vi "air temp subvi remote.vi"(0 "Boolean in":refnum<vi>, 1 "reference 3":refnum<vi>, 2 "reference 11":refnum<vi>, 3 "reference 4":refnum<vi>, 4 "reference 10":refnum<vi>, 5 "reference 5":refnum<vi>, 6 "reference 6":refnum<vi>, 8 "reference 12":refnum<vi>, 9 "reference 7":refnum<vi>, 10 "reference 2":refnum<vi>, 11 "reference 8":refnum<vi>, 12 "reference":refnum<vi>, 13 "reference 9":refnum<vi>, 14 "reference 14":refnum<vi>, 16 "Numeric":dbl) -> ()   [LabVIEW 2018]
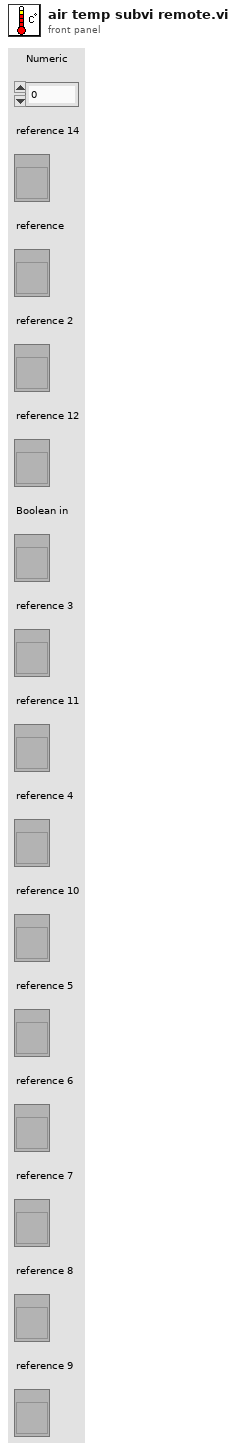
[diagram p1: front panel]
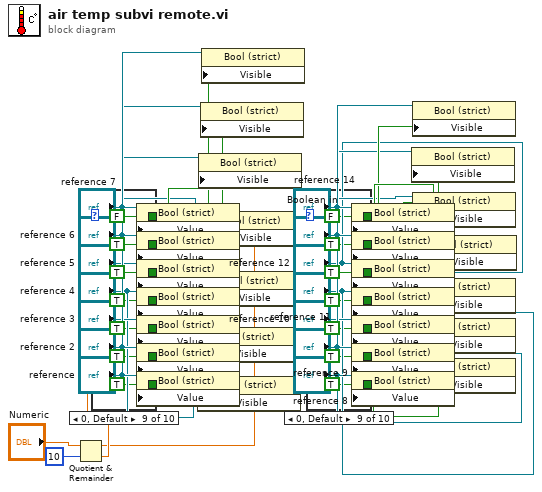
[diagram p0: block diagram]
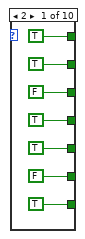
[diagram p2: hidden frame]
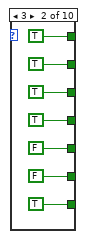
[diagram p3: hidden frame]
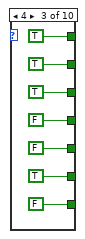
[diagram p4: hidden frame]
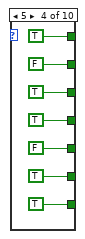
[diagram p5: hidden frame]
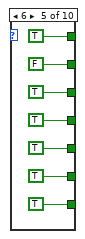
[diagram p6: hidden frame]
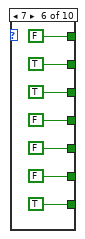
[diagram p7: hidden frame]
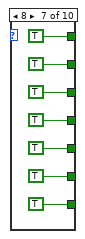
[diagram p8: hidden frame]
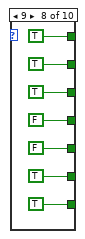
[diagram p9: hidden frame]
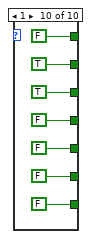
[diagram p10: hidden frame]
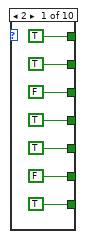
[diagram p11: hidden frame]
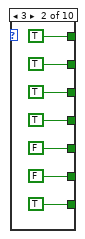
[diagram p12: hidden frame]
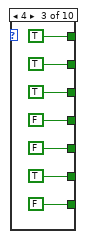
[diagram p13: hidden frame]
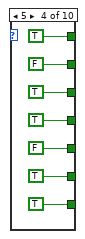
[diagram p14: hidden frame]
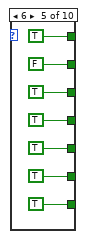
[diagram p15: hidden frame]
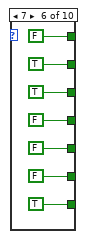
[diagram p16: hidden frame]
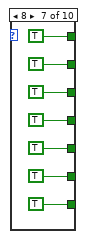
[diagram p17: hidden frame]
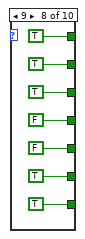
[diagram p18: hidden frame]
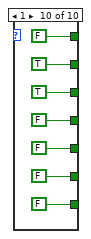
[diagram p19: hidden frame]
diagram:
  n1 = Quotient & Remainder(x="Numeric", y=10) -> (x-y*floor(x/y)=w16:dbl, floor(x/y)=w17:dbl)
  n2 = case shown="0, Default" w17 {
    tunnel: [TRUE TRUE FALSE TRUE TRUE TRUE TRUE TRUE TRUE FALSE] -> w25
    tunnel: [FALSE FALSE TRUE TRUE TRUE FALSE TRUE TRUE TRUE FALSE] -> w26
    tunnel: [TRUE FALSE FALSE FALSE TRUE FALSE TRUE FALSE TRUE FALSE] -> w27
    tunnel: [TRUE TRUE FALSE TRUE TRUE FALSE TRUE FALSE TRUE FALSE] -> w28
    tunnel: [FALSE TRUE TRUE TRUE TRUE TRUE TRUE TRUE TRUE TRUE] -> w29
    tunnel: [TRUE TRUE TRUE FALSE FALSE TRUE TRUE TRUE TRUE TRUE] -> w30
    tunnel: [TRUE TRUE TRUE TRUE TRUE FALSE TRUE TRUE FALSE FALSE] -> w31
    frame 2 {
    }
    frame 3 {
    }
    frame 4 {
    }
    frame 5 {
    }
    frame 6 {
    }
    frame 7 {
    }
    frame 8 {
    }
    frame 9 {
    }
    frame 0, Default {
    }
    frame 1 {
    }
  }
  n3 = property class="Bool (strict)"(reference="reference 7", "Value"=w31) -> ()  [unwired: 1 in, 2 out]
  n4 = property class="Bool (strict)"(reference="reference 6", "Value"=w30) -> ()  [unwired: 1 in, 2 out]
  n5 = property class="Bool (strict)"(reference="reference 5", "Value"=w29) -> ()  [unwired: 1 in, 2 out]
  n6 = property class="Bool (strict)"(reference="reference 4", "Value"=w28) -> ()  [unwired: 1 in, 2 out]
  n7 = property class="Bool (strict)"(reference="reference 3", "Value"=w27) -> ()  [unwired: 1 in, 2 out]
  n8 = property class="Bool (strict)"(reference="reference 2", "Value"=w26) -> ()  [unwired: 1 in, 2 out]
  n9 = property class="Bool (strict)"(reference="reference", "Value"=w25) -> ()  [unwired: 1 in, 2 out]
  n10 = property on="Property Node" class="Bool (strict)"(reference="reference 5", "Visible"=w29) -> ()  [unwired: 1 in, 2 out]
  n11 = property on="Property Node" class="Bool (strict)"(reference="reference 4", "Visible"=w28) -> ()  [unwired: 1 in, 2 out]
  n12 = property on="Property Node" class="Bool (strict)"(reference="reference 6", "Visible"=w30) -> ()  [unwired: 1 in, 2 out]
  n13 = property on="Property Node" class="Bool (strict)"(reference="reference 2", "Visible"=w26) -> ()  [unwired: 1 in, 2 out]
  n14 = property on="Property Node" class="Bool (strict)"(reference="reference 3", "Visible"=w27) -> ()  [unwired: 1 in, 2 out]
  n15 = property on="Property Node" class="Bool (strict)"(reference="reference", "Visible"=w25) -> ()  [unwired: 1 in, 2 out]
  n16 = property on="Property Node" class="Bool (strict)"(reference="reference 7", "Visible"=w31) -> ()  [unwired: 1 in, 2 out]
  n17 = case shown="0, Default" w16 {
    tunnel: [TRUE TRUE FALSE TRUE TRUE TRUE TRUE TRUE TRUE FALSE] -> w18
    tunnel: [FALSE FALSE TRUE TRUE TRUE FALSE TRUE TRUE TRUE FALSE] -> w19
    tunnel: [TRUE FALSE FALSE FALSE TRUE FALSE TRUE FALSE TRUE FALSE] -> w20
    tunnel: [TRUE TRUE FALSE TRUE TRUE FALSE TRUE FALSE TRUE FALSE] -> w21
    tunnel: [FALSE TRUE TRUE TRUE TRUE TRUE TRUE TRUE TRUE TRUE] -> w22
    tunnel: [TRUE TRUE TRUE FALSE FALSE TRUE TRUE TRUE TRUE TRUE] -> w23
    tunnel: [TRUE TRUE TRUE TRUE TRUE FALSE TRUE TRUE FALSE FALSE] -> w24
    frame 2 {
    }
    frame 3 {
    }
    frame 4 {
    }
    frame 5 {
    }
    frame 6 {
    }
    frame 7 {
    }
    frame 8 {
    }
    frame 9 {
    }
    frame 0, Default {
    }
    frame 1 {
    }
  }
  n18 = property class="Bool (strict)"(reference="reference 14", "Value"=w24) -> ()  [unwired: 1 in, 2 out]
  n19 = property class="Bool (strict)"(reference="Boolean in", "Value"=w23) -> ()  [unwired: 1 in, 2 out]
  n20 = property class="Bool (strict)"(reference="reference 12", "Value"=w22) -> ()  [unwired: 1 in, 2 out]
  n21 = property class="Bool (strict)"(reference="reference 11", "Value"=w21) -> ()  [unwired: 1 in, 2 out]
  n22 = property class="Bool (strict)"(reference="reference 10", "Value"=w20) -> ()  [unwired: 1 in, 2 out]
  n23 = property class="Bool (strict)"(reference="reference 9", "Value"=w19) -> ()  [unwired: 1 in, 2 out]
  n24 = property class="Bool (strict)"(reference="reference 8", "Value"=w18) -> ()  [unwired: 1 in, 2 out]
  n25 = property on="Property Node" class="Bool (strict)"(reference="Boolean in", "Visible"=w23) -> ()  [unwired: 1 in, 2 out]
  n26 = property on="Property Node" class="Bool (strict)"(reference="reference 9", "Visible"=w19) -> ()  [unwired: 1 in, 2 out]
  n27 = property on="Property Node" class="Bool (strict)"(reference="reference 14", "Visible"=w24) -> ()  [unwired: 1 in, 2 out]
  n28 = property on="Property Node" class="Bool (strict)"(reference="reference 12", "Visible"=w22) -> ()  [unwired: 1 in, 2 out]
  n29 = property on="Property Node" class="Bool (strict)"(reference="reference 11", "Visible"=w21) -> ()  [unwired: 1 in, 2 out]
  n30 = property on="Property Node" class="Bool (strict)"(reference="reference 8", "Visible"=w18) -> ()  [unwired: 1 in, 2 out]
  n31 = property on="Property Node" class="Bool (strict)"(reference="reference 10", "Visible"=w20) -> ()  [unwired: 1 in, 2 out]
